vi "Intake Modifications.vi"(1 "Intake Info In":T1, 2 "Cannon vbus":dbl) -> (0 "Intake Info In":T1)   [LabVIEW 2013]
panel:
  in  "t":dbl=1.05
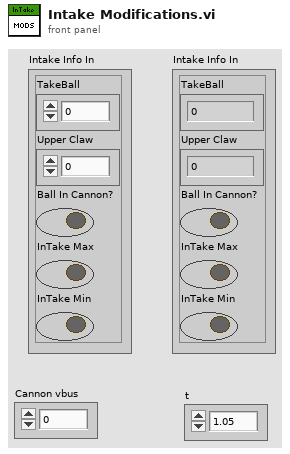
[diagram p1: front panel]
types:
  T1 = cluster{"TakeBall":dbl, "Upper Claw":dbl, "Ball In Cannon?":bool, "InTake Max":bool, "InTake Min":bool}
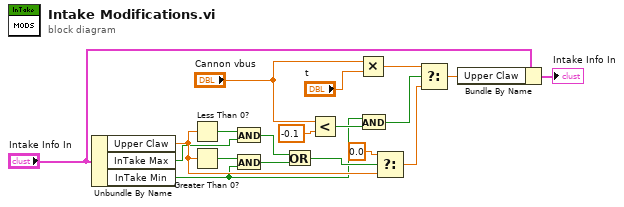
[diagram p0: block diagram]
diagram:
  n1 = Unbundle By Name("Intake Info In") -> ("Upper Claw"=w6:dbl, "InTake Max"=w5:bool, "InTake Min"=w3:bool)
  n2 = Less Than 0?(x=w6) -> (x < 0?=w7:bool)
  n3 = Greater Than 0?(x=w6) -> (x > 0?=w10:bool)
  n4 = And(x=w7, y=w5) -> (x .and. y?=w8:bool)
  n5 = And(x=w10, y=w3) -> (x .and. y?=w9:bool)
  n6 = Or(x=w8, y=w9) -> (x .or. y?=w11:bool)
  n7 = Less?(x="Cannon vbus", y=-0.1) -> (x < y?=w13:bool)
  n8 = Multiply(x="Cannon vbus", y="t") -> (x*y=w16:dbl)
  n9 = And(x=w3, y=w13) -> (x .and. y?=w14:bool)
  n10 = Select(t=0.0, s=w11, f=w6) -> (s? t:f=w17:dbl)
  n11 = Select(t=w16, s=w14, f=w17) -> (s? t:f=w4:dbl)
  n12 = Bundle By Name(cluster="Intake Info In", "Upper Claw"=w4) -> (→"Intake Info In":T1)
